vi "Member Split Names.vi"(8 "error in (no error)":errorcluster, 11 "Search in":refnum<class "Search.lvclass">) -> (0 "error out":errorcluster, 3 "Search out":refnum<class "Search.lvclass">)   [LabVIEW 2020, in "Better Search.lvlib" / "Search.lvclass"]
uses:
  Search.lvclass
  Search.lvclass/Search.ctl
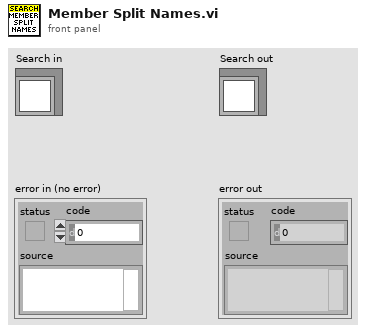
[diagram p1: front panel]
types:
  T1 = typedef "Better Search.lvlib/Type Reflection Item.ctl" = cluster{"Parent":i32, "Depth":i32, "Children":i32[], "Skip":bool, "Name":string, "Type":variant, "TypeID":string}
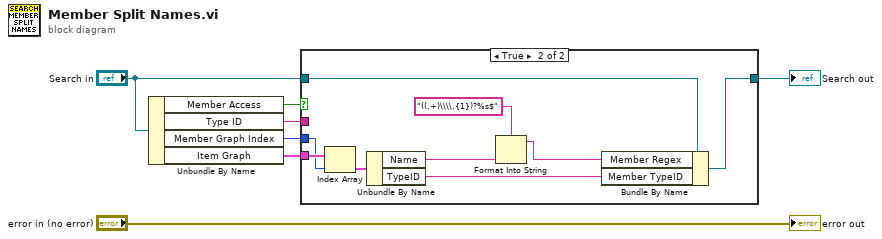
[diagram p0: block diagram]
diagram:
  n1 = Unbundle By Name("Search in") -> ("Member Access"=w4:bool, "Type ID"=w3:string, "Member Graph Index"=w2:i32, "Item Graph"=w1:T1[])
  n2 = case shown="True" w4 {
    tunnel: "Search in" -> [w8 w17]
    tunnel: [w8 w16] -> w5
    tunnel: w3 -> [_ _]
    tunnel: w2 -> [_ w13]
    tunnel: w1 -> [_ w14]
    frame False {
    }
    frame True {
      n3 = Index Array(array=w14, index=w13) -> (element=w12:T1)
      n4 = Unbundle By Name(w12) -> ("Name"=w10:string, "TypeID"=w15:string)
      n5 = Format Into String(format string="((.+)\\\\.{1})?%s$", w10) -> (resulting string=w9:string)  [unwired: 2 in, 1 out]
      n6 = Bundle By Name(cluster=w17, "Member Regex"=w9, "Member TypeID"=w15) -> (w16:refnum<class "Search.lvclass">)
    }
  }
  "Search out" <- w5
  "error out" <- "error in (no error)"
